vi "Sync Config from Instr.vi"(8 "error in (no error)":errorcluster, 11 "Instrument Actor in":refnum<class "Instrument Actor.lvclass">) -> (0 "error out":errorcluster, 3 "Instrument Actor out":refnum<class "Instrument Actor.lvclass">)   [LabVIEW 2021, in "Instrument Actor.lvclass"]
uses:
  Instrument Actor.lvclass
  <vilib>/Utility/Data Type/Type Definitions/Data Type.ctl
  <vilib>/Utility/Data Type/Type Definitions/Type Definition Info.ctl
  Instrument Actor.lvclass/Instrument Actor.ctl
  Read Instrument driver.vi
  Write Instrument driver.vi
  NHMFL_Core/Libraries/Instruments/Instrument Driver/Instrument Driver.lvclass
  <vilib>/Utility/Data Type/NI_Data Type.lvlib
panel:
  out "type definition info":T1
  out "type definition":bool
  out "name":string
  out "type":T2
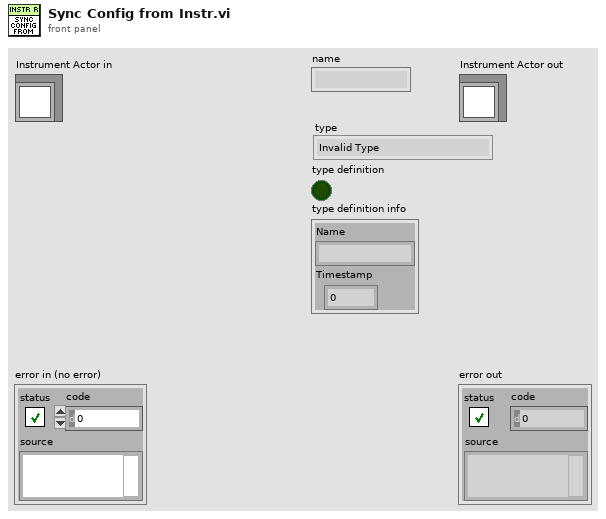
[diagram p1: front panel]
types:
  T1 = typedef "NI_Data Type.lvlib/Type Definition Info.ctl" = cluster{"Name":string, "Timestamp":u32}
  T2 = typedef "NI_Data Type.lvlib/Data Type.ctl" = enum8{"Invalid Type", "Void", "I8", "I16", "I32", "I64", "U8", "U16", "U32", "U64", "Single Float", "Double Float", "Extended Float", "Single Complex", "Double Complex", "Extended Complex", "Enum U8", "Enum U16", "Enum U32", "Enum U64", "Single Float With Unit", "Double Float With Unit", "Extended Float With Unit", "Single Complex with Unit", "Double Complex with Unit", "Extended Complex with Unit", "Boolean", "String", "Path", "Picture", "Tag", "Array", "Cluster", "Variant", "LV Variant", "Waveform", "Timestamp", "Digital Waveform", "Digital Data", "ExpressData", "Refnum", "External Data", "VI", "Poly VI", "LabVIEW Class Instance", "Fixed Point", "Set Collection", "Map Collection"}
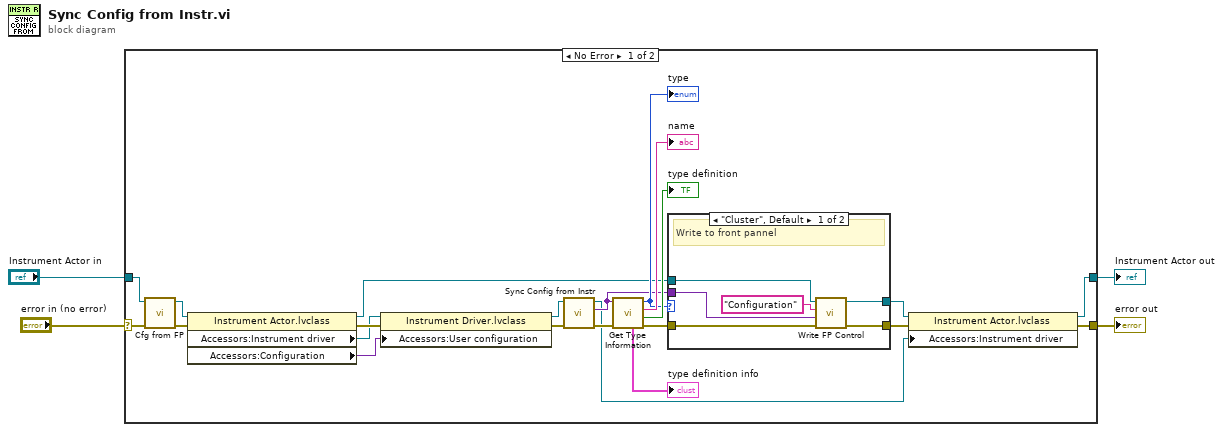
[diagram p0: block diagram]
diagram:
  n1 = case shown="No Error" "error in (no error)" {
    selector: "error in (no error)" -> [w9 w36]
    tunnel: [w16 w36] -> w3
    tunnel: [w14 w35] -> w1
    tunnel: "Instrument Actor in" -> [w12 w35]
    frame No Error {
      n2 = call-dynamic "Cfg from FP.vi"("error in (no error)"=w9, "Measure Object in"=w12) -> ("error out"=w10:errorcluster, "Measure Object out"=w11:refnum<class "Instrument Actor.lvclass">)  [unwired: 8 in]
      n3 = property class="Instrument Actor.lvclass"(reference=w11, error in=w10) -> (reference out=w20:refnum<class "Instrument Actor.lvclass">, error out=w26:errorcluster, "Accessors:Instrument driver"=w7:refnum<class "Instrument Driver.lvclass">, "Accessors:Configuration"=w5:variant)
      n4 = property class="Instrument Driver.lvclass"(reference=w7, error in=w26, "Accessors:User configuration"=w5) -> (reference out=w6:refnum<class "Instrument Driver.lvclass">, error out=w8:errorcluster)
      n5 = call-dynamic "Sync Config from Instr.vi"("error in (no error)"=w8, "Instrument Driver in"=w6) -> ("error out"=w22:errorcluster, "Variant"=w18:variant, "Instrument Driver out"=w13:refnum<class "Instrument Driver.lvclass">)  [unwired: 7 in]
      n6 = call <vilib>:"Get Type Information.vi"("error in (no error)"=w22, "variant"=w18) -> ("error out"=w19:errorcluster, "type definition"=→"type definition":bool, "name"=→"name":string, "type"=w21:T2, "type definition info"=→"type definition info":T1)  [unwired: 5 in]
      "type" <- w21
      n7 = case shown="\"Cluster\", Default" w21 {
        tunnel: w20 -> [w32 w33]
        tunnel: w19 -> [w30 w34]
        tunnel: w18 -> [w29 _]
        tunnel: [w28 w34] -> w17
        tunnel: [w27 w33] -> w15
        frame "Cluster", Default {
          # "Write to front pannel"
          n8 = call-dynamic "Write FP Control.vi"("error in (no error)"=w30, "Control Value"=w29, "Control Name"="Configuration", "Measure Object in"=w32) -> ("error out"=w28:errorcluster, "Measure Object out"=w27:refnum<class "Instrument Actor.lvclass">)  [unwired: 6 in]
        }
        frame "Invalid Type", "Void" {
          # "Skip if not defined (default parent behaviour)"
        }
      }
      n9 = property class="Instrument Actor.lvclass"(reference=w15, error in=w17, "Accessors:Instrument driver"=w13) -> (reference out=w14:refnum<class "Instrument Actor.lvclass">, error out=w16:errorcluster)
    }
    frame Error {
    }
  }
  "error out" <- w3
  "Instrument Actor out" <- w1
